vi "Get Question for Candidate.vi"(0 "element":T1={"ID"="", "Name"="", "Email"="", "Start Time"=timestamp(0 s since 1904-01-01), "State"=enum."LoggedIn", "Answer[]"=[], "ActiveQuestionID"=""}, 5 "QID":string, 11 "error in (no error)":errorcluster) -> (4 "element 2":T1={"ID"="", "Name"="", "Email"="", "Start Time"=timestamp(0 s since 1904-01-01), "State"=enum."LoggedIn", "Answer[]"=[], "ActiveQuestionID"=""}, 15 "error out":errorcluster)   [LabVIEW 2014, in "Coding Platform.lvlib"]
uses:
  Coding Platform.lvlib
  Typedefs/Candidate.ctl
  Typedefs/Candidate State.ctl
  Typedefs/Answer Info.ctl
  Typedefs/Answer State.ctl
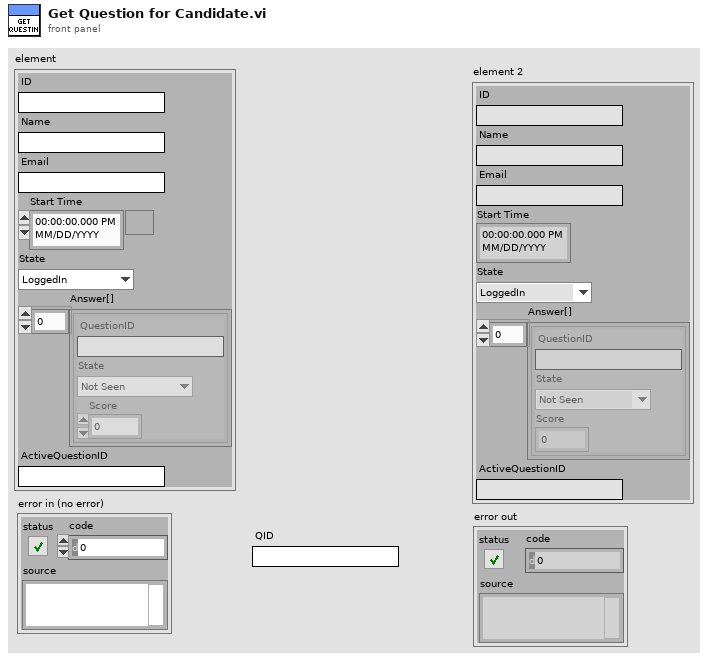
[diagram p1: front panel]
types:
  T1 = typedef "Coding Platform.lvlib/Candidate.ctl" = cluster{"ID":string, "Name":string, "Email":string, "Start Time":timestamp, "State":T2, "Answer[]":T3[], "ActiveQuestionID":string}
  T2 = typedef "Coding Platform.lvlib/Candidate State.ctl" = enum16{"Unknown", "LoggedIn", "In Test", "Completed Test"}
  T3 = typedef "Coding Platform.lvlib/Answer Info.ctl" = cluster{"QuestionID":string, "State":T4, "Score":u64}
  T4 = typedef "Coding Platform.lvlib/Answer State.ctl" = enum16{"Not Seen", "In Progress", "Completed"}
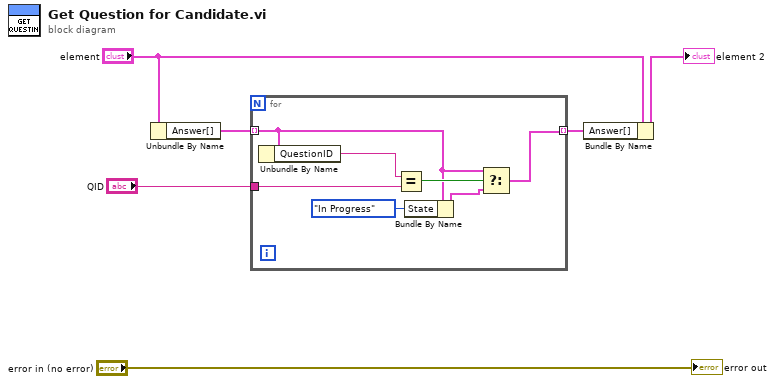
[diagram p0: block diagram]
diagram:
  n1 = Unbundle By Name("element") -> ("Answer[]"=w2:T3[])
  n2 = for {
    tunnel: [w10] -> w3 mode=indexing
    tunnel: w2 -> [w9] mode=indexing
    tunnel: "QID" -> [w12]
    n3 = Unbundle By Name(w9) -> ("QuestionID"=w13:string)
    n4 = Equal?(x=w13, y=w12) -> (x = y?=w11:bool)
    n5 = Bundle By Name(cluster=w9, "State"=Answer_State."In Progress") -> (w8:T3)
    n6 = Select(t=w9, s=w11, f=w8) -> (s? t:f=w10:T3)
  }
  n7 = Bundle By Name(cluster="element", "Answer[]"=w3) -> (→"element 2":T1)
  "error out" <- "error in (no error)"
